vi "HTTP Spool Response.vi"(8 "error in (no error)":errorcluster, 9 "Message (optional)":string, 10 "Timeout (ms)":i32=-1, 11 "connection ID":refnum<k5>) -> (0 "error out":errorcluster, 1 "Content-Length":i32, 2 "HTTP REQUEST/RESPONSE":string, 3 "connection ID out":refnum<k5>, 4 "HTTP Body":string, 5 "HTTP Headers":string, 6 "Time to receive response":u32, 7 "timeout expired?":bool)   [LabVIEW 2011]
panel:
  out "numLoops":i32
  in  "bytes to read":i32=128
  out "Header-Length":i32
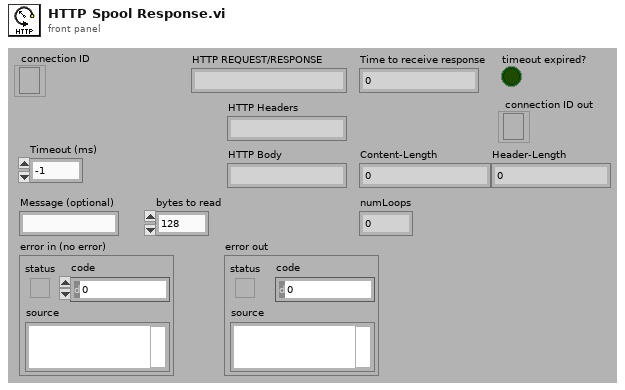
[diagram p1: front panel]
types:
  T1 = enum16{"Standard", "Buffered", "CRLF", "Immediate"}
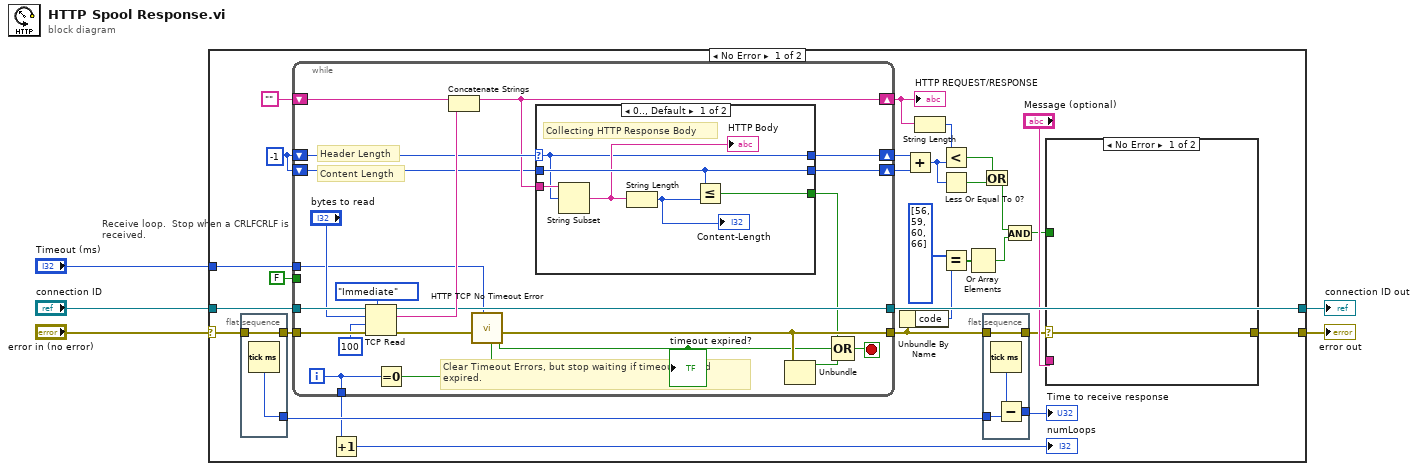
[diagram p0: block diagram]
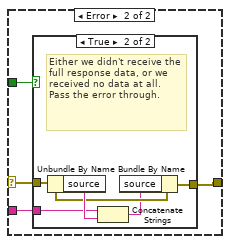
[diagram p2: hidden frame]
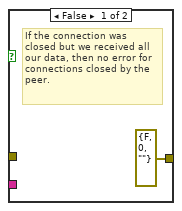
[diagram p3: hidden frame]
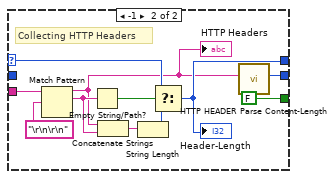
[diagram p4: hidden frame]
diagram:
  n1 = case shown="No Error" "error in (no error)" {
    selector: "error in (no error)" -> [w28 w90]
    tunnel: [w32 w89] -> w5
    tunnel: [w27 w90] -> w4
    tunnel: "connection ID" -> [w30 w89]
    tunnel: "Timeout (ms)" -> [w24 _]
    frame No Error {
      w21 = -1 ("timeout ms (25000)")
      n2 = flat-sequence {
        tunnel: w28 -> [w45]
        tunnel: [w45] -> _
        tunnel: [w44] -> w31
        frame #0 {
          n3 = Tick Count (ms)() -> (millisecond timer value=w44:u32)
        }
      }
      n4 = while "Receive loop.  Stop when a CRLFCRLF is received." {
        tunnel: w28 -> [w67]
        shift-left: "" -> [w49]
        shift-right: [w53] -> w19
        tunnel: [w63] -> w12
        tunnel: w30 -> [w65]
        tunnel: [w60] -> w32
        tunnel: [w62] -> w29
        tunnel: w24 -> [w47]
        shift-right: [w52] -> w16
        shift-left: w21 -> [w54]
        shift-right: [w50] -> w17
        shift-left: w21 -> [w51]
        tunnel: FALSE -> [_]
        i -> [w62]
        stop <- w55 stop-if-true
        # "Content Length"
        # "Header Length"
        # "Clear Timeout Errors, but stop waiting if timeout period expired."
        n5 = TCP Read(connection ID=w65, bytes to read="bytes to read", error in (no error)=w67, 7:T1."Immediate" ("mode (standard)"), 9:100 ("timeout ms (25000)")) -> (connection ID out=w60:refnum<k5>, data out=w66:string, error out=w64:errorcluster)
        n6 = Equal To 0?(x=w62) -> (x = 0?=w61:bool)
        n7 = Concatenate Strings(w49, w66) -> (w53:string)
        n8 = call "HTTP TCP No Timeout Error.vi"("Restart Timeout?"=w61, "Timeout ms (-1)"=w47, "error in (no error)"=w64) -> ("timeout expired?"=w56:bool, "error out"=w63:errorcluster)  [unwired: 7 in]
        "timeout expired?" <- w56
        n9 = case shown="0.., Default" w54 {
          selector: w54 -> [w68 w80]
          tunnel: [w73 FALSE] -> w58
          tunnel: w53 -> [w70 w82]
          tunnel: [w68 w76] -> w52
          tunnel: w51 -> [w71 _]
          tunnel: [w71 w75] -> w50
          frame 0.., Default {
            # "Collecting HTTP Response Body"
            n10 = String Subset(string=w70, offset (0)=w68) -> (substring=w69:string)  [unwired: 1 in]
            "HTTP Body" <- w69
            n11 = String Length(string=w69) -> (length=w72:i32)
            "Content-Length" <- w72
            n12 = Less Or Equal?(x=w71, y=w72) -> (x <= y?=w73:bool)
          }
          frame -1 {
            # "Collecting HTTP Headers"
            n13 = Match Pattern(string=w82, regular expression="\r\n\r\n") -> (before substring=w74:string, match substring=w78:string)  [unwired: 3 out]
            "HTTP Headers" <- w74
            n14 = Empty String/Path?(string/path=w78) -> (empty?=w81:bool)
            n15 = Concatenate Strings(w74, w78) -> (w77:string)
            n16 = String Length(string=w77) -> (length=w79:i32)
            n17 = Select(t=w80, s=w81, f=w79) -> (s? t:f=w76:i32)
            "Header-Length" <- w76
            n18 = call "HTTP HEADER Parse Content-Length.vi"("HTTP HEADERS"=w74) -> ("Content-Length"=w75:i32)  [unwired: 10 in]
          }
        }
        n19 = Unbundle(w63) -> ("status"=w57:bool)  [unwired: 2 out]
        n20 = Compound Arithmetic op=OR(w58, w56, w57) -> (w55:bool)
      }
      "HTTP REQUEST/RESPONSE" <- w19
      n21 = Increment(x=w29) -> (x+1=→"numLoops":i32)
      n22 = Unbundle By Name(w12) -> ("code"=w15:i32)
      n23 = Add(x=w16, y=w17) -> (x+y=w6:i32)
      n24 = String Length(string=w19) -> (length=w18:i32)
      n25 = Less?(x=w18, y=w6) -> (x < y?=w9:bool)
      n26 = Less Or Equal To 0?(x=w6) -> (x <= 0?=w7:bool)
      n27 = Equal?(x=i32[] [56, 59, 60, 66], y=w15) -> (x = y?=w14:bool[])
      n28 = Or Array Elements(Boolean array=w14) -> (logical OR=w10:bool)
      n29 = Or(x=w9, y=w7) -> (x .or. y?=w8:bool)
      n30 = flat-sequence {
        tunnel: w12 -> [w85]
        tunnel: w31 -> [w87]
        tunnel: [w86] -> w23
        tunnel: [w85] -> _
        frame #0 {
          n31 = Tick Count (ms)() -> (millisecond timer value=w88:u32)
          n32 = Subtract(x=w88, y=w87) -> (x-y=w86:u32)
        }
      }
      n33 = And(x=w8, y=w10) -> (x .and. y?=w13:bool)
      n34 = case shown="No Error" w12 {
        selector: w12 -> [w33 w36]
        tunnel: [w33 w35] -> w27
        tunnel: "Message (optional)" -> [_ w37]
        tunnel: w13 -> [_ w34]
        frame No Error {
        }
        frame Error {
          n35 = case shown="True" w34 {
            tunnel: w37 -> [_ w42]
            tunnel: w36 -> [_ w41]
            tunnel: [errorcluster {"status"=FALSE, "code"=0, "source"=""} ("error IO") w40] -> w35
            frame False {
              # "If the connection was closed but we received all our data, then no error for connections closed by the peer."
            }
            frame True {
              # "Either we didn't receive the full response data, or we received no data at all.  Pass the error through."
              n36 = Unbundle By Name(w41) -> ("source"=w43:string)
              n37 = Concatenate Strings(w42, w43) -> (w39:string)
              n38 = Bundle By Name(cluster=w41, "source"=w39) -> (w40:errorcluster)
            }
          }
        }
      }
      "Time to receive response" <- w23
    }
    frame Error {
    }
  }
  "error out" <- w4
  "connection ID out" <- w5
